vi "RUSHDriveTrain.vi"(0 "Servo Positions":T1, 5 "Low Gear + Brake":bool, 7 "Low Gear":bool, 9 "LeftJoystick":dbl, 11 "RightJoystick":dbl) -> (4 "Braking Servo":dbl, 6 "Left Drive":dbl, 8 "Right Drive":dbl, 10 "Left Servo":dbl, 15 "Right Servo":dbl)   [LabVIEW 2012]
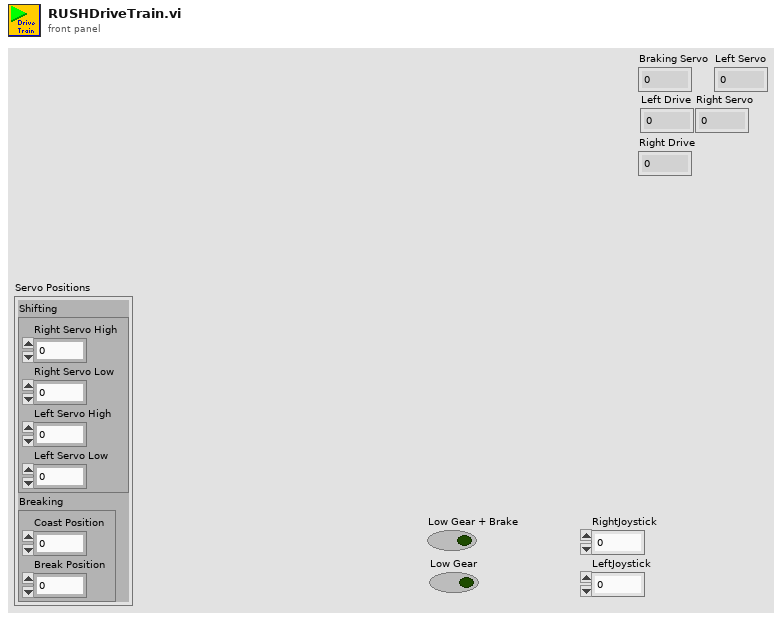
[diagram p1: front panel]
types:
  T1 = cluster{"Shifting":cluster{"Right Servo High":dbl, "Right Servo Low":dbl, "Left Servo High":dbl, "Left Servo Low":dbl}, "Breaking":cluster{"Coast Position":dbl, "Break Position":dbl}}
  T2 = cluster{"Right Servo High":dbl, "Right Servo Low":dbl, "Left Servo High":dbl, "Left Servo Low":dbl}
  T3 = cluster{"Coast Position":dbl, "Break Position":dbl}
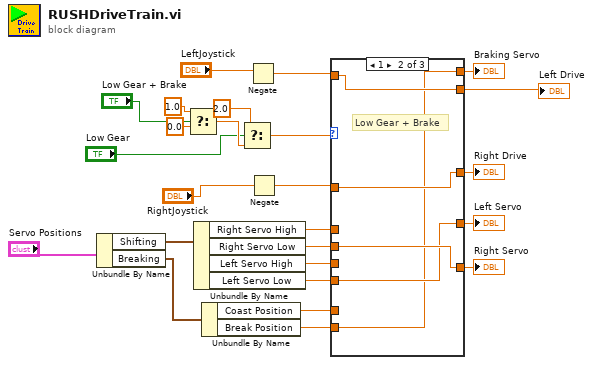
[diagram p0: block diagram]
diagram:
  n1 = Unbundle By Name("Servo Positions") -> ("Shifting"=w14:T2, "Breaking"=w12:T3)
  n2 = Select(t=1.0, s="Low Gear + Brake", f=0.0 ("t")) -> (s? t:f=w23:dbl)
  n3 = Unbundle By Name(w14) -> ("Right Servo High"=w6:dbl, "Right Servo Low"=w7:dbl, "Left Servo High"=w8:dbl, "Left Servo Low"=w9:dbl)
  n4 = Unbundle By Name(w12) -> ("Coast Position"=w10:dbl, "Break Position"=w11:dbl)
  n5 = Select(t=2.0, s="Low Gear", f=w23) -> (s? t:f=w21:dbl)
  n6 = Negate(x="LeftJoystick") -> (-x=w20:dbl)
  n7 = Negate(x="RightJoystick") -> (-x=w19:dbl)
  n8 = case shown="1" w21 {
    tunnel: w19 -> [w30 w35 w40]
    tunnel: [w30 w35 w40] -> w3
    tunnel: [w29 w34 w39] -> w4
    tunnel: [w27 w32 w37] -> w2
    tunnel: [w26 w33 w38] -> w1
    tunnel: w20 -> [w29 w34 w39]
    tunnel: [w28 w31 w36] -> w5
    tunnel: w11 -> [_ w31 _]
    tunnel: w10 -> [w28 _ w36]
    tunnel: w9 -> [_ w32 w37]
    tunnel: w8 -> [w27 _ _]
    tunnel: w7 -> [_ w33 w38]
    tunnel: w6 -> [w26 _ _]
    frame 0, Default {
      # "High Gear"
    }
    frame 1 {
      # "Low Gear + Brake"
    }
    frame 2 {
      # "Low Gear"
    }
  }
  "Braking Servo" <- w5
  "Left Drive" <- w4
  "Right Drive" <- w3
  "Left Servo" <- w2
  "Right Servo" <- w1
